vi "Process X Y to angle.vi"(3 "Point position":cluster{"Width":dbl, "High":dbl}) -> (1 "Angle (rad)":dbl)   [LabVIEW 2017]
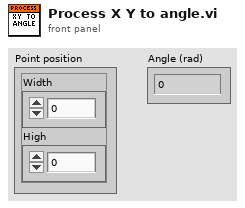
[diagram p1: front panel]
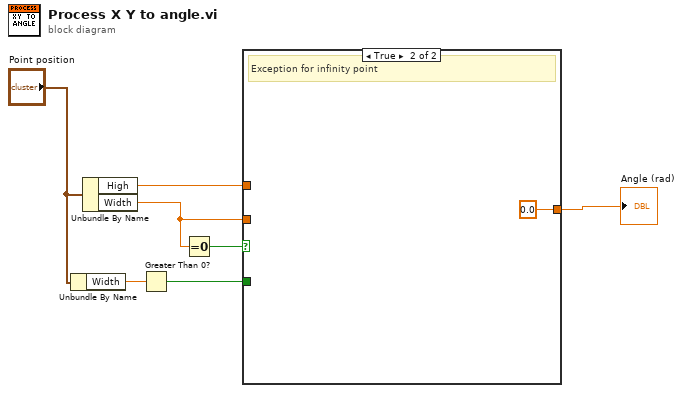
[diagram p0: block diagram]
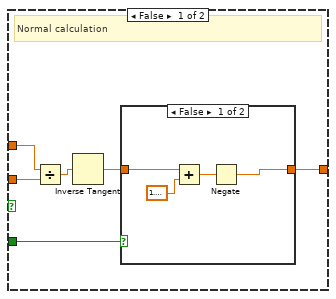
[diagram p2: hidden frame]
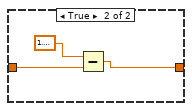
[diagram p3: hidden frame]
diagram:
  n1 = Unbundle By Name("Point position") -> ("Width"=w4:dbl)
  n2 = Unbundle By Name("Point position") -> ("High"=w3:dbl, "Width"=w2:dbl)
  n3 = Greater Than 0?(x=w4) -> (x > 0?=w5:bool)
  n4 = Equal To 0?(x=w2) -> (x = 0?=w1:bool)
  n5 = case shown="True" w1 {
    tunnel: [w13 0.0] -> w6
    tunnel: w5 -> [w12 _]
    tunnel: w3 -> [w11 _]
    tunnel: w2 -> [w8 _]
    frame False {
      # "Normal calculation"
      n6 = Divide(x=w11, y=w8) -> (x/y=w10:dbl)
      n7 = Inverse Tangent(1:w10) -> (0:w9:dbl)
      n8 = case shown="False" w12 {
        tunnel: [w14 w20] -> w13
        tunnel: w9 -> [w17 w18]
        frame False {
          n9 = Add(x=w17, y=1.5707963267948966) -> (x+y=w15:dbl)
          n10 = Negate(x=w15) -> (-x=w14:dbl)
        }
        frame True {
          n11 = Subtract(x=1.5707963267948966, y=w18) -> (x-y=w20:dbl)
        }
      }
    }
    frame True {
      # "Exception for infinity point"
    }
  }
  "Angle (rad)" <- w6
